vi "Acquire Data using 5772 without DRAM_sim_temp.vi"() -> ()   [LabVIEW 2011]
uses:
  <vilib>/Platform/TimedLoop/XDataNode/timing_clust.ctl
  <vilib>/Platform/TimedLoop/XDataNode/nitl_modes.ctl
  <vilib>/Platform/TimedLoop/XDataNode/wakeup.ctl
  <vilib>/rvi/FIFO/Fifo_Resource/nirvififoEmulationSetSize.vi
  <vilib>/rvi/DataTransferAndStorage/Container/Common/niFpgaContainerGetUniqueNameForEmu.vi
  <vilib>/Platform/TimedLoop/XDataNode/XDataNode.xnode
  <vilib>/rvi/FXPMathLib/basic elements/FxpDiscreteDelay/XNode/nifxpmath_DiscreteDelay.xnode
  <vilib>/rvi/DataTransferAndStorage/Container/XNode/niFpgaContainer.xnode
  <vilib>/rvi/FIFO/Fifo_Resource/nirvififoEmulationWrite.vi
  <vilib>/Platform/TimedLoop/XDataNode/XDNodeRunTimeDep.lvlib
  <instrlib>/FlexRIO/Libraries/Acquisition Engine/Acquisition Engine.lvlib
panel:
  out "count":u32
  out "NumSamplesAcquired":u32
  out "Host FIFO Timed Out?":bool
  in  "Host Trigger":bool=TRUE
  in  "Trigger Type":T1(ring)=enum."Software Trigger"
  in  "acq.Post Trig":u32=10
  in  "acq.Pre Trig":u32=2 min=2 step=1
  in  "acq.Record Count":u32=1
  in  "acq.Initiate":bool=TRUE
  # "Digitial Trigger Input:\nPXI_Trig0 or DIO 0 on CB Front Panel"
  # "Interactive Mode Instructions\n1) Run the Emulation Mode VI for Stimulus\n1) Click on acq.Initiate, First to False and Then to True\n2) Click on Host Trigger"
  # "Trigger Selection"
  # "Acquisition Engine"
  # "Status"
  # "Record Retrieval"
  # "Memory Configuration"
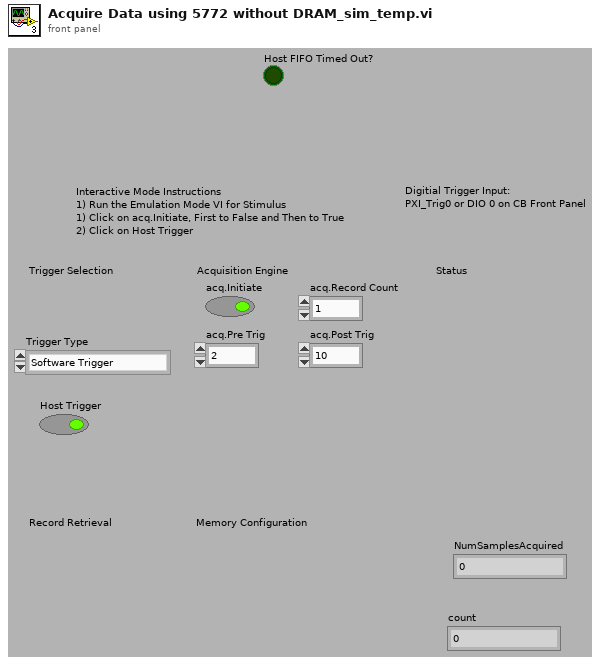
[diagram p1: front panel]
types:
  T1 = enum8{"Immediate Trigger", "Software Trigger", "External Digital Trigger", "Analog Trigger"}
  T2 = typedef "XDNodeRunTimeDep.lvlib/timing_clust.ctl" = cluster{"Expected End [f-1]":u64, "Actual End [f-1]":u64, "Finished Late? [f-1]":bool, "Expected End [i-1]":u64, "Actual End [i-1]":u64, "Finished Late? [i-1]":bool, "Expected Start [i]":u64, "Actual Start [i]":u64, "Expected Start [f]":u64, "Actual Start [f]":u64, "Source Name":string, "Structure Name":string, "Period":i64, "Deadline":i64, "Offset":i64, "Start":i64, "Priority":i32, "Timeout":i32, "Mode":T3, "Wakeup Reason":T4, "Error":errorcluster, "Source Type":string, "Secondary Source Type":string, "Global End Time":u64, "Global Start Time":u64, "Frame Duration":u64, "Iteration Duration":u64, "Assigned CPU":i32, "I/O Scan Engine Mode":u32}
  T3 = typedef "XDNodeRunTimeDep.lvlib/nitl_modes.ctl" = enum32{"No Change", "Process missed periods, maintain original phase", "Discard missed periods, maintain original phase", "Process missed periods, ignore original phase", "Discard missed periods, ignore original phase"}
  T4 = typedef "XDNodeRunTimeDep.lvlib/wakeup.ctl" = enum32{"Normal", "Aborted", "Asynchronous wakeup", "Timing source error", "Timed loop error", "Timeout"}
  T5 = typedef "acqEngineStates v1.ctl" = cluster{"Triggered":bool, "TrigArmed":bool, "RdyForArm":bool, "Reserved":bool}
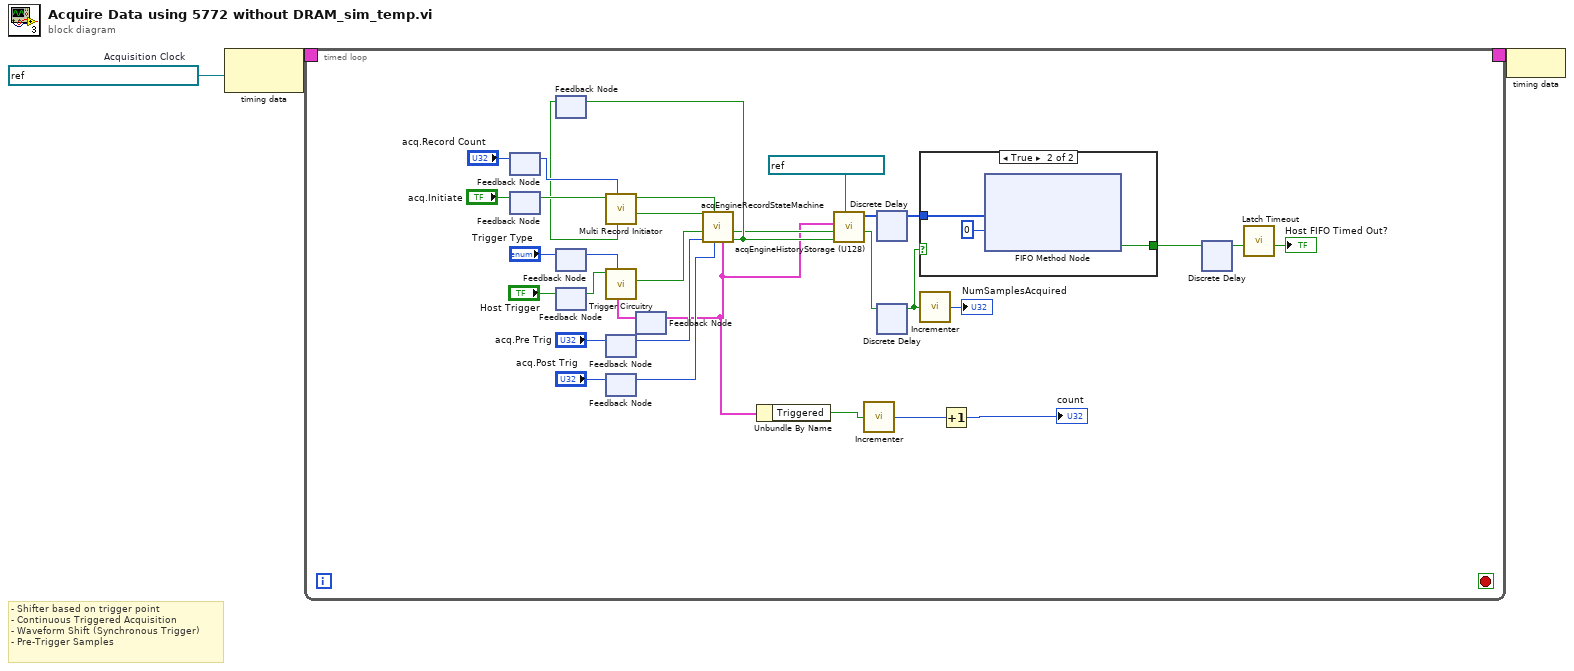
[diagram p0: block diagram]
diagram:
  w1 = refnum<k21> "IO Module Clock 0"  # Acquisition Clock
  # "- Shifter based on trigger point\n- Continuous Triggered Acquisition\n- Waveform Shift (Synchronous Trigger)\n- Pre-Trigger Samples"
  n1 = node-c288(w1) -> (w3:T2)
  n2 = timed-loop {
    timing: w3 -> [_]
    timing-out: [_] -> w2
    stop <- _ stop-if-true
    n3 = feedback-in #1("acq.Record Count") -> ()
    n4 = feedback #1() -> (w28:u32)  [unwired: 1 in]
    n5 = feedback-in #2("acq.Initiate") -> ()
    n6 = feedback #2() -> (w27:bool)  [unwired: 1 in]
    n7 = feedback #3() -> (w10:bool)  [unwired: 1 in]
    n8 = feedback #4() -> (w25:T1)  [unwired: 1 in]
    n9 = feedback-in #4("Trigger Type") -> ()
    n10 = feedback-in #5("Host Trigger") -> ()
    n11 = feedback #5() -> (w24:bool)  [unwired: 1 in]
    n12 = call <instrlib>:"Multi Record Initiator.vi"("Record Completed"=w10, "acq.Record Count"=w28, "acq.Initiate"=w27) -> ("send start trigger"=w9:bool, "send acq.Initiate"=w11:bool)  [unwired: 7 in]
    n13 = feedback-in #6("acq.Pre Trig") -> ()
    n14 = feedback #6() -> (w23:u32)  [unwired: 1 in]
    n15 = feedback-in #7("acq.Post Trig") -> ()
    n16 = feedback #7() -> (w22:u32)  [unwired: 1 in]
    n17 = feedback #8() -> (w30:T5)  [unwired: 1 in]
    n18 = call <userlib>:"Trigger Circuitry.vi"("State Machine State"=w30, "Trigger Type"=w25, "Software Trigger from Host"=w24) -> ("Trigger Out"=w31:bool)  [unwired: 7 in, 1 out]
    n19 = call <instrlib>:"acqEngineRecordStateMachine.vi"("acq.Post Trig"=w22, "acq.Initiate"=w11, "acq.Pre Trig"=w23, "Trig"=w31, "StartTrig"=w9) -> ("PostTrigComplete"=w21:bool, "AcqInProgress"=w8:bool, "states"=w4:T5)  [unwired: 4 in]
    n20 = feedback-in #3(w21) -> ()
    n21 = feedback-in #8(w4) -> ()
    n22 = Unbundle By Name(w4) -> ("Triggered"=w6:bool)
    n23 = call "acqEngineHistoryStorage (U128).vi"("FIFO Out"=refnum<k21> "HistoryFIFOU128", "PostTrigComplete"=w21, "AcqInProgress"=w8, "states"=w4) -> ("valid"=w18:bool, "Output Data"=w19:i16[])  [unwired: 5 in, 1 out]
    n24 = call <userlib>:"Incrementer.vi"("INC?"=w6) -> ("count"=w7:u32)  [unwired: 4 in]
    n25 = xnode "Discrete Delay"("D"=w19) -> ("Q"=w14:i16[])
    n26 = xnode "Discrete Delay"("D"=w18) -> ("Q"=w13:bool)
    n27 = case shown="True" w13 {
      tunnel: w14 -> [_ w38]
      tunnel: [_ w36] -> w15
      frame False {
      }
      frame True {
        n28 = xnode ("FIFO Method Node")("Element"=w38, "Timeout"=0) -> ("Timed Out?"=w36:bool)  [unwired: 1 in, 1 out]
      }
    }
    n29 = call <userlib>:"Incrementer.vi"("INC?"=w13) -> ("count"=→"NumSamplesAcquired":u32)  [unwired: 4 in]
    n30 = Increment(x=w7) -> (x+1=→"count":u32)
    n31 = xnode "Discrete Delay"("D"=w15) -> ("Q"=w16:bool)
    n32 = call <userlib>:"Latch Timeout.vi"("Timeout?"=w16) -> ("Ever Timed Out?"=→"Host FIFO Timed Out?":bool)  [unwired: 10 in]
  }
  n33 = node-c288(w2) -> ()
